vi "Read RT Dataset.vi"(8 "error in (no error)":errorcluster, 10 "Connected System":string, 11 "MiniGUI in":refnum<class "MiniGUI.lvclass">) -> (0 "error out":errorcluster, 3 "MiniGUI out":refnum<class "MiniGUI.lvclass">)   [LabVIEW 2019, in "MiniGUI.lvlib" / "MiniGUI.lvclass"]
uses:
  MiniGUI.lvclass
  MiniGUI.lvclass/MiniGUI.ctl
  <vilib>/regexp/Match Regular Expression.xnode
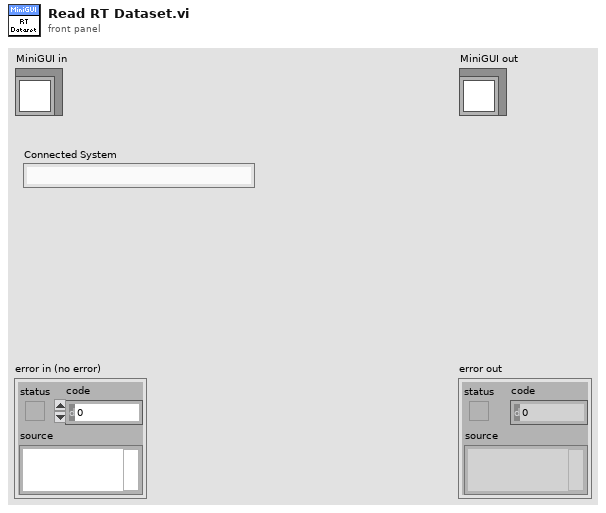
[diagram p1: front panel]
types:
  T1 = enum8{"Enabled", "Disabled", "Disabled and Grayed Out"}
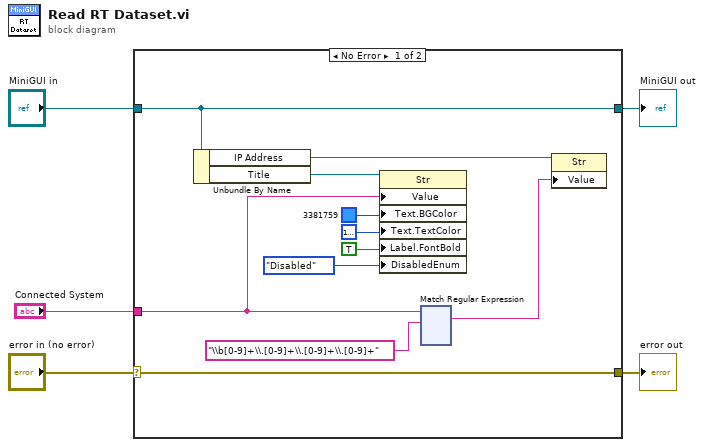
[diagram p0: block diagram]
diagram:
  n1 = case shown="No Error" "error in (no error)" {
    selector: "error in (no error)" -> [w6 w132]
    tunnel: [w6 w132] -> w4
    tunnel: [w16 w131] -> w2
    tunnel: "MiniGUI in" -> [w16 w131]
    tunnel: "Connected System" -> [w12 _]
    frame No Error {
      n2 = Unbundle By Name(w16) -> ("IP Address"=w15:refnum<vi>, "Title"=w14:refnum<vi>)
      n3 = property class="Str"(reference=w14, "Value"=w12, "Text.BGColor"=u32 3381759 ("Text.Text Colors:BG Color"), "Text.TextColor"=u32 16777225 ("Text.Text Colors:Text Color"), "Label.FontBold"=TRUE ("Text.Font:Bold"), "DisabledEnum"=T1."Disabled" ("Disabled")) -> ()  [unwired: 1 in, 2 out]
      n4 = xnode ("Match Regular Expression")("input string"=w12, "regular expression"="\\b[0-9]+\\.[0-9]+\\.[0-9]+\\.[0-9]+") -> ("whole match"=w7:string)  [unwired: 4 in, 4 out]
      n5 = property class="Str"(reference=w15, "Value"=w7) -> ()  [unwired: 1 in, 2 out]
    }
    frame Error {
    }
  }
  "error out" <- w4
  "MiniGUI out" <- w2
